vi "Auto Align.vi"(10 "Right Side?":bool, 11 "Target Data":T1) -> (2 "Aligned?":bool, 3 "Motor Out":cluster{"output":dbl, dbl})   [LabVIEW 2011]
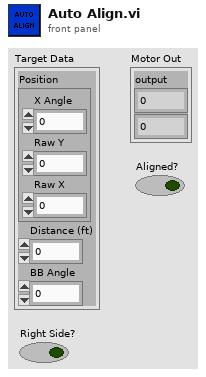
[diagram p1: front panel]
types:
  T1 = cluster{"Position":cluster{"X Angle":dbl, "Raw Y":dbl, "Raw X":dbl}, "Distance (ft)":dbl, "BB Angle":dbl}
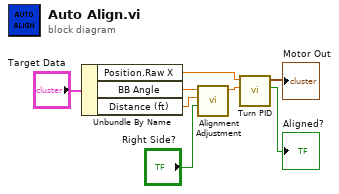
[diagram p0: block diagram]
diagram:
  n1 = Unbundle By Name("Target Data") -> ("Position.Raw X"=w3:dbl, "BB Angle"=w2:dbl, "Distance (ft)"=w1:dbl)
  n2 = call "Alignment Adjustment.vi"("Right Side of Field?"="Right Side?", "Distance"=w1, "BB Angle"=w2) -> ("X Setpoint"=w4:dbl)  [unwired: 8 in]
  n3 = call "Turn PID.vi"("Setpoint X"=w4, "Current X"=w3) -> ("Aligned?"=→"Aligned?":bool, "Motor Out"=→"Motor Out":cluster{"output":dbl, dbl})  [unwired: 8 in]
